vi "LDF Get Sch Frame Name.vi"(7 "pFrameName":string, 9 "index":i32, 10 "pSchName":string, 11 "LDFHandle":u64) -> (2 "pSchName out":string, 3 "function return":i32, 5 "pFrameName out":string)   [LabVIEW 2010, in "ldf_parser.lvlib"]
doc: "int WINAPI LDF_GetSchFrameName(long long LDFHandle, char* pSchName, int index, char* pFrameName);"
uses:
  ldf_parser.lvlib
  USB2XXX/trunk/USB2XXX/USB2XXX/vs2019/Release/USB2XXX.dll
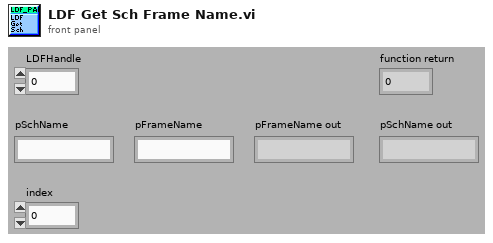
[diagram p1: front panel]
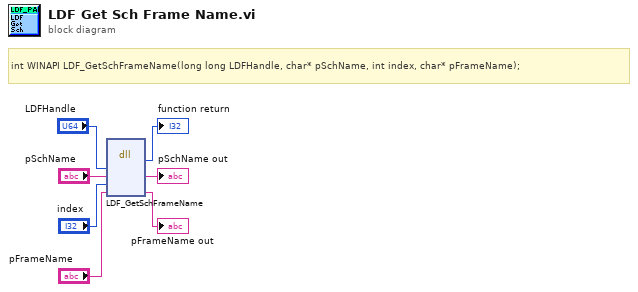
[diagram p0: block diagram]
diagram:
  # "int WINAPI LDF_GetSchFrameName(long long LDFHandle, char* pSchName, int index, char* pFrameName);"
  n1 = dll-call lib="E:/Projects/USB2XXX/trunk/USB2XXX/USB2XXX/vs2019/Release/USB2XXX.*" fn="LDF_GetSchFrameName"("LDFHandle"="LDFHandle", "pSchName"="pSchName", "index"="index", "pFrameName"="pFrameName") -> (→"function return":i32, "pSchName"=→"pSchName out":string, "pFrameName"=→"pFrameName out":string)  [unwired: 5 in, 2 out]
